vi "Autotuning PID Online.vi"() -> ()   [LabVIEW 2023]
doc: "This example demonstrates how to use Advanced PID autotuning VI where you can change the autotuning algorithm while you run the VI."
uses:
  <vilib>/addons/control/pid/NI_PID_autopid.lvlib
panel:
  out "tuning completed?":bool
  in  "Tab Control":enum32{"Instructions"}(tab)
  in  "Instructions":string="Overview: This example demonstrates how to use Advanced PID autotuning VI where you can change the autotuning algorithm while the VI is running.\nInstructions:\n1. Run the VI and wait until the process variable (PV) reaches near setpoint (SP).\n2.  On the PID Autotuning Design section, select the type of algorithm, type of controller and excitation amplitude for the 'open loop step response'. Then, press Autotune to start the process.\n3.  When the tuned PID gains do not change anymore or the tuning completed? flashes, the identification is done and you can accept new gains by pressing Accept gain and that will transfer the new gain to PID Gains.\n4. Click Autotune to go back to the automatic control. You can try different options and repeat this process.\n5. Click Stop to stop the VI.\n"
  in  "setpoint\nweighting\n(gamma)":dbl(knob) scale=0.0..1.0
  in  "Set \nInitial Gain?":bool
  in  "Initial PID Gains":T1={"proportional gain (Kc)"=2.1923418207514507, "integral time (Ti, min)"=0.006000000284984708, "derivative time (Td, min)"=0.0} {"derivative time (Td, min)" format="%#.6g"; "integral time (Ti, min)" format="%#.6g"; "proportional gain (Kc)" format="%#.6g"}
  in  "Automatic":bool=TRUE
  in  "setpoint\nweighting\n(beta)":dbl(knob)=3.8231445459877658 scale=0.0..1.0
  in  "Reinitialize":bool
  in  "autotuning parameters":T2={"technique"=2, "controller type"=1, "control specification"=0, "amplitude"=1.0} {"amplitude" format="%.2f"; "control specification" items=["fast", "normal", "slow"]; "controller type" items=["P", "PI", "PID"]; "technique" items=["Step Open Loop", "Step Closed Loop", "Relay", "PID Relay"]}
  out "MV":dbl(graph)=18.823532635520305
  in  "Accept Gain?":bool
  out "tuned PID gains":T1={"proportional gain (Kc)"=15.221889907608013, "integral time (Ti, min)"=0.002027201803862475, "derivative time (Td, min)"=0.0002815558060920104} {"derivative time (Td, min)" format="%#.6g"; "integral time (Ti, min)" format="%#.6g"; "proportional gain (Kc)" format="%#.6g"}
  in  "Autotune":bool
  in  "SP:":dbl(slide)=47.05882352941177 min=0.0 max=0.0 scale=0.0..100.0
  in  "MV:":dbl(slide)=18.823532635520305 scale=-100.0..100.0
  out "PV:":dbl(slide)=47.05872530934063 scale=0.0..100.0
  in  "PID Gains":T1={"proportional gain (Kc)"=15.221889907608013, "integral time (Ti, min)"=0.002027201803862475, "derivative time (Td, min)"=0.0002815558060920104} {"derivative time (Td, min)" format="%#.6g"; "integral time (Ti, min)" format="%#.6g"; "proportional gain (Kc)" format="%#.6g"}
  in  "Sampling Time dt (s)":dbl=0.05 min=0.001 step=0.01 format="%#.3p"
  in  "Stop":bool
  out "SP and PV":cluster{"initial PV":dbl, "SP1:":dbl}(graph)={"initial PV"=47.05872530934063, "SP1:"=47.05882352941177}
  # "Proportional-Integral-Derivative (PID) Controller"
  # "PID Autotuning Design"
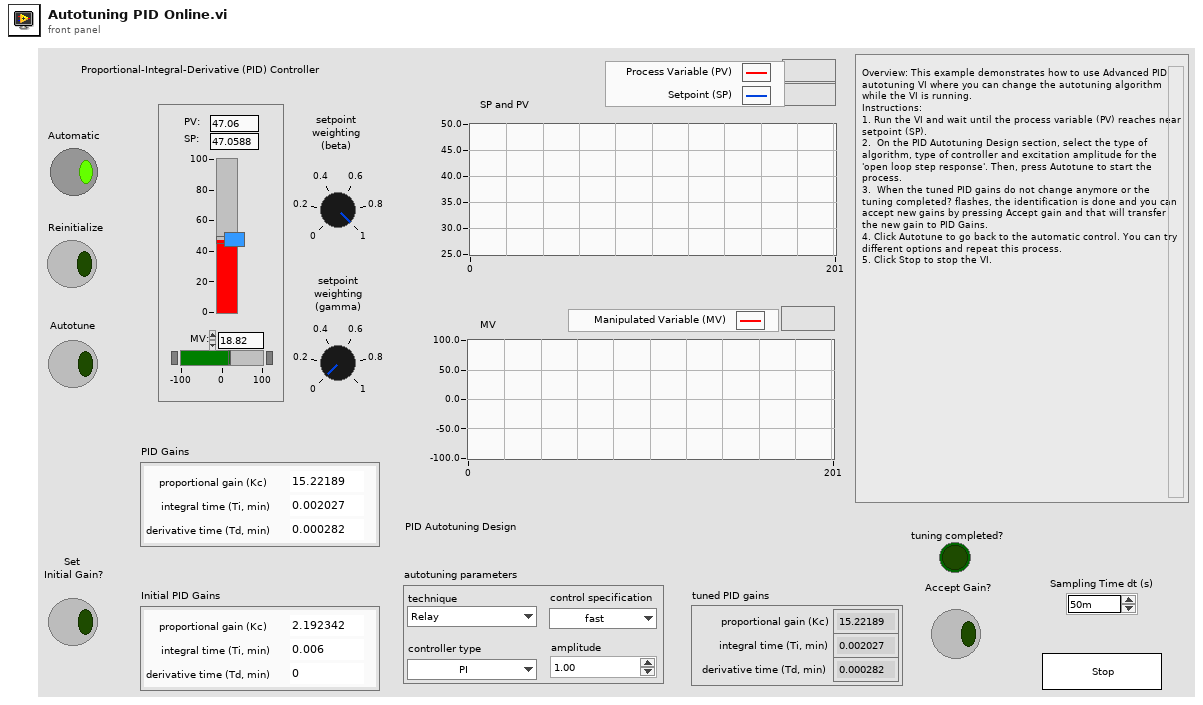
[diagram p1: front panel]
types:
  T1 = cluster{"proportional gain (Kc)":dbl, "integral time (Ti, min)":dbl, "derivative time (Td, min)":dbl}
  T2 = cluster{"technique":u16, "controller type":u16, "control specification":u16, "amplitude":dbl}
  T3 = cluster{"static gain":dbl, "lag (s)":dbl, "deadtime (s)":dbl, "load":dbl, "deadband":dbl, "sensor noise":dbl, "initial PV":dbl, "plant noise":dbl}
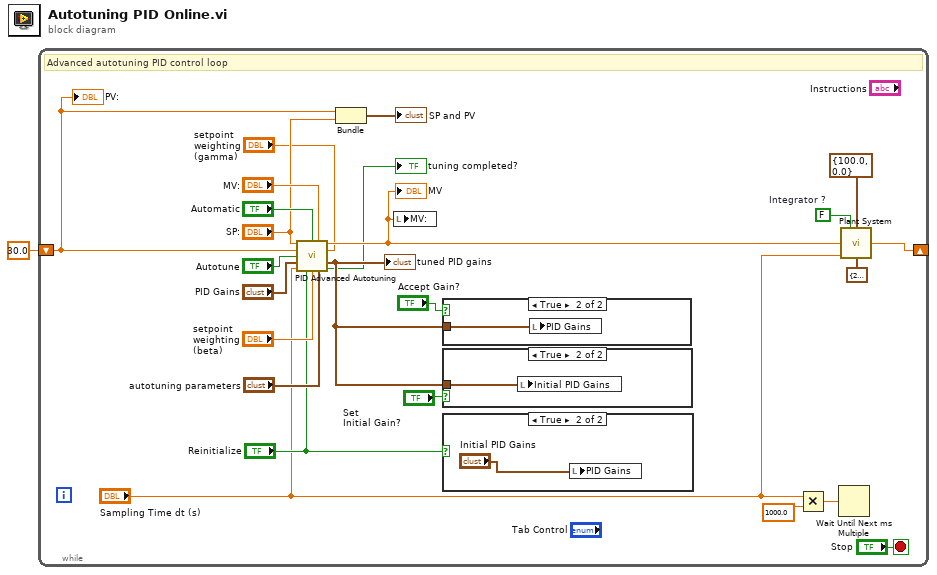
[diagram p0: block diagram]
diagram:
  n1 = while {
    shift-left: 30.0 ("initial PV") -> [w16]
    shift-right: [w24] -> _
    stop <- "Stop" stop-if-true
    w11 = FALSE  # Integrator ?
    # "Advanced autotuning PID control loop"
    n2 = call <vilib>:"PID Advanced Autotuning.vi"("setpoint"="SP:", "auto? (F)"="Automatic", "manual control"="MV:", "process variable"=w16, "gamma"="setpoint\nweighting\n(gamma)", "autotune? (F)"="Autotune", "PID gains"="PID Gains", "dt (s)"="Sampling Time dt (s)", "reinitialize? (F)"="Reinitialize", "beta"="setpoint\nweighting\n(beta)", "autotuning parameters"="autotuning parameters") -> ("output"=w21:dbl, "tuned PID gains"=w5:T1, "tuning completed?"=→"tuning completed?":bool)  [unwired: 2 in]
    "MV" <- w21
    "tuned PID gains" <- w5
    n3 = Bundle("initial PV"=w16, "SP:"="SP:") -> (→"SP and PV":cluster{"initial PV":dbl, "SP:":dbl})  [unwired: 1 in]
    n4 = local write "MV:"(w21) -> ()
    n5 = case shown="True" "Accept Gain?" {
      tunnel: w5 -> [_ w28]
      frame False {
      }
      frame True {
        n6 = local write "PID Gains"(w28) -> ()
      }
    }
    n7 = case shown="True" "Set \nInitial Gain?" {
      tunnel: w5 -> [_ w27]
      frame False {
      }
      frame True {
        n8 = local write "Initial PID Gains"(w27) -> ()
      }
    }
    n9 = case shown="True" "Reinitialize" {
      frame False {
      }
      frame True {
        n10 = local write "PID Gains"("Initial PID Gains") -> ()
      }
    }
    n11 = Multiply(x="Sampling Time dt (s)", y=1000.0 ("Simulation Time (times)")) -> (x*y=w8:dbl)
    n12 = Wait Until Next ms Multiple(millisecond multiple=w8) -> ()  [unwired: 1 out]
    n13 = call "Plant System.vi"("Integrator ?"=w11, "output saturation range"=cluster{"output high":dbl, "output low":dbl} {"output high"=100.0, "output low"=0.0}, "Plant Input"=w21, "dt (s)"="Sampling Time dt (s)", "process parameters"=T3 {"static gain"=2.5, "lag (s)"=2.5, "deadtime (s)"=0.001, "load"=0.0, "deadband"=0.0, "sensor noise"=0.0, "initial PV"=0.0, "plant noise"=0.0}) -> ("Plant Output"=w24:dbl)  [unwired: 10 in]
    "PV:" <- w16
  }
